vi "TDK-Lambda Z Output Volt Arbitrary Waveform.vi"() -> ()   [LabVIEW 2020]
doc: "This example shows how to configure a transient mode and set up triggering.\n1. Set Property Communication Parameters\n2. Set Required Output Values and then RUN"
uses:
  TDK-Lambda Z.lvlib
panel:
  in  "Configuration":T1={"Address"=6, "Baud Rate"=9600, "Language Selector"=1} {"Language Selector" items=["GEN", "SCPI"]; "Baud Rate" items=["1200"=1200, "2400"=2400, "4800"=4800, "9600"=9600, "19200"=19200, "38400"=38400, "57600"=57600, "115200"=115200]}
  in  "Reset(True)":bool=TRUE
  in  "Continuous Trigger (F: Off)":bool
  in  "Time Points":dbl[](array[numeric]) format="%#_6f"
  in  "Value Points":dbl[](array[numeric]) format="%#_6f"
  in  "Step & Counter":cluster{"Step (0: Once)":u16, "Counter (1)":i32}={"Step (0: Once)"=0, "Counter (1)"=1} {"Counter (1)" min=1 max=9999 step=1; "Step (0: Once)" items=["Once", "Auto"]}
  in  "Current Limit (0A)":dbl format="%.4f"
  in  "Voltage Limit (0V)":dbl format="%.4f"
  in  "VISA resource name":refnum<visa-resource-name>
  # "(c) 2014-2015 TDK-Lambda.  ALL RIGHTS RESERVED."
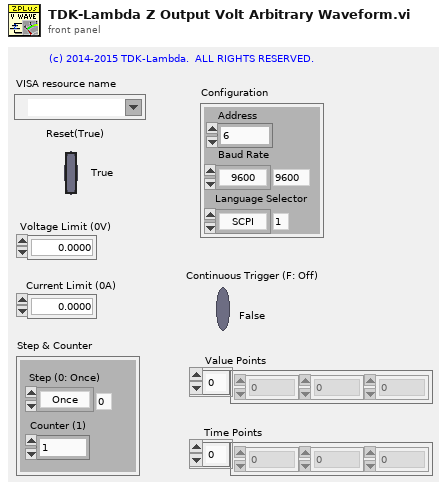
[diagram p1: front panel]
types:
  T1 = cluster{"Address":i16, "Baud Rate":u32, "Language Selector":i16}
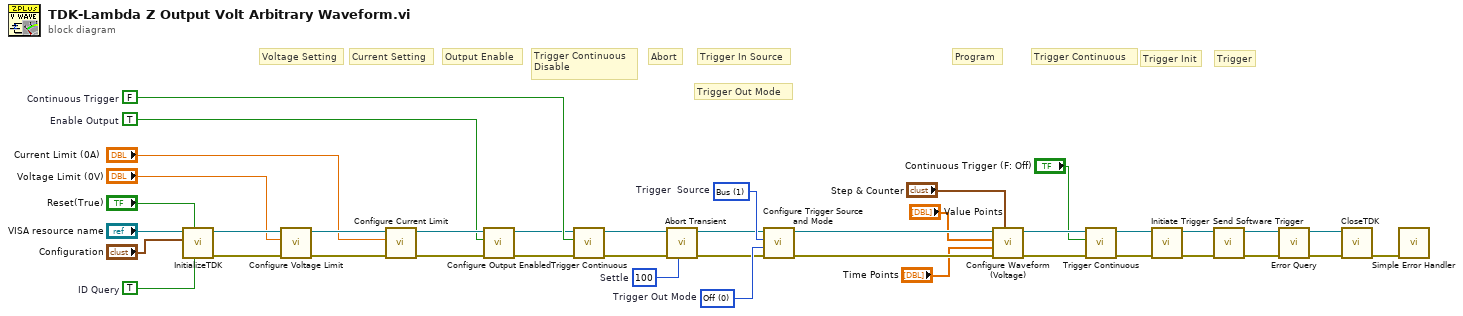
[diagram p0: block diagram]
diagram:
  w18 = FALSE  # Continuous Trigger
  w19 = u16 0 items=["Off", "Trigger", "FSTR"]  # Trigger Out Mode
  w20 = u16 1 items=["External", "Bus"]  # Trigger  Source
  w21 = TRUE  # Enable Output
  w22 = u32 100  # Settle
  w23 = TRUE  # ID Query
  # "Trigger Continuous"
  # "Trigger Continuous\nDisable"
  # "Trigger"
  # "Trigger Init"
  # "Program"
  # "Trigger Out Mode"
  # "Trigger In Source"
  # "Abort"
  # "Output Enable"
  # "Current Setting"
  # "Voltage Setting"
  n1 = call "InitializeTDK.vi"("ID Query (True)"=w23, "Reset(True)"="Reset(True)", "Configuration"="Configuration", "VISA resource name"="VISA resource name") -> ("error out"=w37:errorcluster, "VISA resource name out"=w40:refnum<visa-resource-name>)  [unwired: 6 in]
  n2 = call "Configure Voltage Limit.vi"("error in (no error)"=w37, "Voltage Limit (0V)"="Voltage Limit (0V)", "VISA resource name"=w40) -> ("error out"=w36:errorcluster, "VISA resource name out"=w39:refnum<visa-resource-name>)  [unwired: 7 in]
  n3 = call "Configure Current Limit.vi"("error in (no error)"=w36, "Current Limit (0A)"="Current Limit (0A)", "VISA resource name"=w39) -> ("error out"=w35:errorcluster, "VISA resource name out"=w38:refnum<visa-resource-name>)  [unwired: 7 in]
  n4 = call "Configure Output Enabled.vi"("error in (no error)"=w35, "Enable Output (F: Off)"=w21, "VISA resource name"=w38) -> ("error out"=w11:errorcluster, "VISA resource name out"=w12:refnum<visa-resource-name>)  [unwired: 7 in]
  n5 = call "Trigger Continuous.vi"("error in (no error)"=w11, "Continuous Trigger (F: Off)"=w18, "VISA resource name"=w12) -> ("error out"=w9:errorcluster, "VISA resource name out"=w10:refnum<visa-resource-name>)  [unwired: 7 in]
  n6 = call "Abort Transient.vi"("Settle (1mS)"=w22, "error in (no error)"=w9, "VISA resource name"=w10) -> ("error out"=w7:errorcluster, "VISA resource name out"=w8:refnum<visa-resource-name>)  [unwired: 7 in]
  n7 = call "Configure Trigger Source and Mode.vi"("error in (no error)"=w7, "Trigger Out Mode (0: Off)"=w19, "Trigger  Source (0: External)"=w20, "VISA resource name"=w8) -> ("error out"=w33:errorcluster, "VISA resource name out"=w34:refnum<visa-resource-name>)  [unwired: 6 in]
  n8 = call "Configure Waveform (Voltage).vi"("Step & Counter"="Step & Counter", "error in (no error)"=w33, "Time Points"="Time Points", "Value Points"="Value Points", "VISA resource name"=w34) -> ("error out"=w17:errorcluster, "VISA resource name out"=w16:refnum<visa-resource-name>)  [unwired: 5 in]
  n9 = call "Trigger Continuous.vi"("error in (no error)"=w17, "Continuous Trigger (F: Off)"="Continuous Trigger (F: Off)", "VISA resource name"=w16) -> ("error out"=w14:errorcluster, "VISA resource name out"=w15:refnum<visa-resource-name>)  [unwired: 7 in]
  n10 = call "Initiate Trigger.vi"("error in (no error)"=w14, "VISA resource name"=w15) -> ("error out"=w31:errorcluster, "VISA resource name out"=w32:refnum<visa-resource-name>)  [unwired: 8 in]
  n11 = call "Send Software Trigger.vi"("error in (no error)"=w31, "VISA resource name"=w32) -> ("error out"=w30:errorcluster, "VISA resource name out"=w2:refnum<visa-resource-name>)  [unwired: 8 in]
  n12 = call "Error Query.vi"("error in (no error)"=w30, "VISA resource name"=w2) -> ("error out"=w3:errorcluster, "VISA resource name out"=w1:refnum<visa-resource-name>)  [unwired: 6 in, 2 out]
  n13 = call "CloseTDK.vi"("error in (no error)"=w3, "VISA resource name"=w1) -> ("error out"=w4:errorcluster)  [unwired: 9 in]
  n14 = call "Simple Error Handler.vi"("error in (no error)"=w4) -> ()  [unwired: 4 in, 5 out]
